vi "Main_PIDTune.vi"() -> ()   [LabVIEW 2015]
doc: "View output from heater including temperature, heater status, temp set point, heater set, and current PWM output (as controlled by PID)."
uses:
  <vilib>/Instr/_visa.llb/VISA Configure Serial Port (Instr).vi
panel:
  out "concatenated string":string
  in  "PID values Set":dbl[](array[numeric])
  out "PID values":dbl[](array[numeric])
  out "PWM":i32
  out "On/Off Set":bool
  out "Measurement History":waveform(dbl)(graph)
  out "Set Point FB":i32 caption="Temp Set Point (C)"
  out "Heater Status":bool
  out "Temp (C)":dbl
  in  "Set Point (C)":i32 caption="Temp Set Point (C)" min=0 max=40
  in  "Heater":bool
  in  "String":string
  in  "Send":bool
  in  "stop":bool
  out "Time of Read":string
  out "Serial Buffer":string
  in  "VISA resource name":refnum<visa-resource-name>
  # "Fluid Heater Control"
  # "Feedback"
  # "Setpoint"
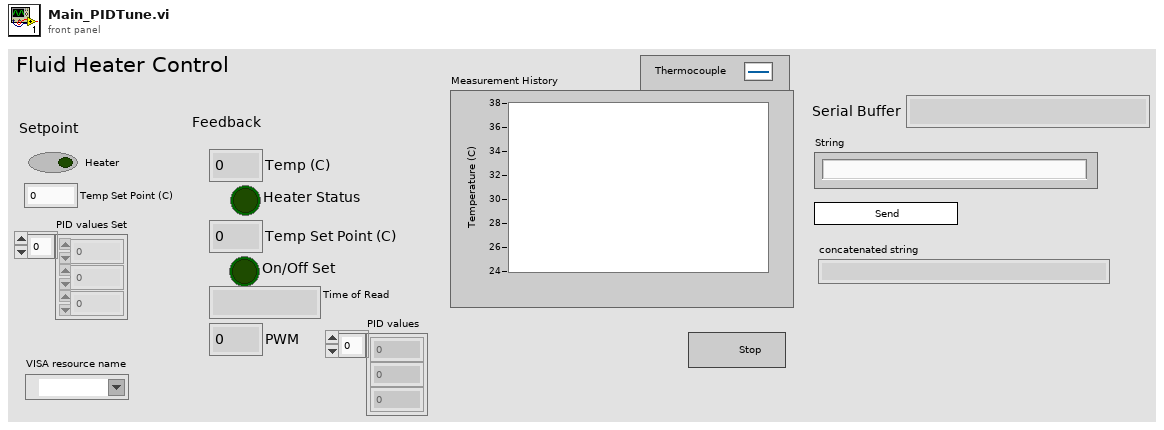
[diagram p1: front panel]
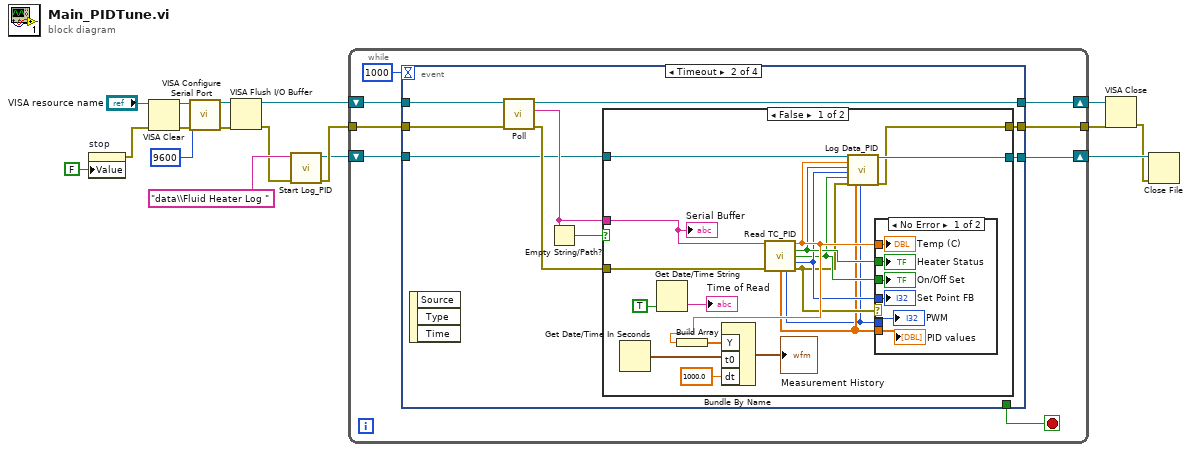
[diagram p0: block diagram]
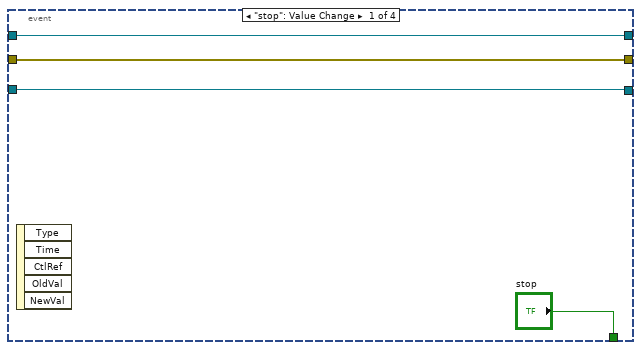
[diagram p2: hidden frame]
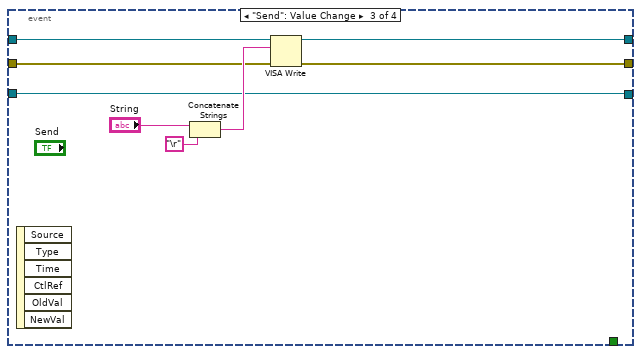
[diagram p5: hidden frame]
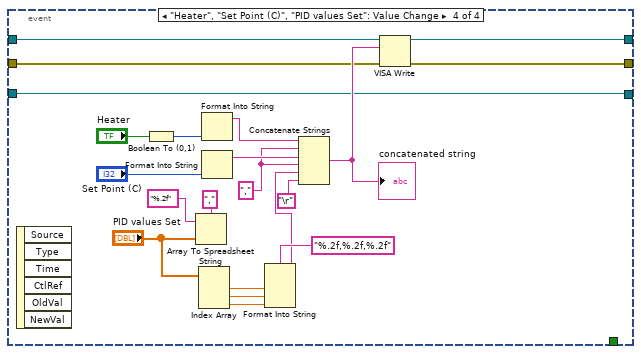
[diagram p6: hidden frame]
diagram:
  n1 = property on="stop" class="Bool (strict)"("Value"=FALSE ("stop")) -> (error out=w8:errorcluster)  [unwired: 2 in, 1 out]
  n2 = VISA Clear(VISA resource name="VISA resource name", error in (no error)=w8) -> (VISA resource name out=w13:refnum<visa-resource-name>, error out=w16:errorcluster)
  n3 = call-poly "VISA Configure Serial Port"("VISA resource name"=w13, "baud rate (9600)"=u32 9600, "error in (no error)"=w16) -> ("VISA resource name out"=w12:refnum<visa-resource-name>, "error out"=w17:errorcluster)  [unwired: 11 in]
  n4 = VISA Flush I/O Buffer(VISA resource name=w12, error in (no error)=w17) -> (VISA resource name out=w11:refnum<visa-resource-name>, error out=w5:errorcluster)  [unwired: 1 in]
  n5 = call "Start Log_PID.vi"("Error In"=w5, "Log Prefix"="data\\Fluid Heater Log ") -> ("Error Out"=w4:errorcluster, "refnum out"=w3:refnum<file>)  [unwired: 8 in]
  n6 = while {
    tunnel: w4 -> [w22]
    shift-right: [w21] -> w10
    shift-left: w11 -> [w23]
    tunnel: [w20] -> w9
    shift-right: [w18] -> w2
    shift-left: w3 -> [w19]
    stop <- w25 stop-if-true
    n7 = event shown="[1] Timeout" {
      selector: _ -> [_ _ _ _]
      dyn-events: _ -> [_ _ _ _]
      timeout: 1000 -> [_ _ _ _]
      tunnel: ["stop" _ _ _] -> w25
      tunnel: w23 -> [w28 w36 w69 w87]
      tunnel: w22 -> [w27 w35 w67 w86]
      tunnel: [w28 w34 w68 w85] -> w21
      tunnel: [w27 w30 w66 w84] -> w20
      tunnel: w19 -> [w26 w32 w65 w83]
      tunnel: [w26 w31 w65 w83] -> w18
      event "stop": Value Change {
        n8 = event-data() -> ()  [unwired: 1 in, 5 out]
      }
      event Timeout {
        n9 = event-data() -> ()  [unwired: 1 in, 3 out]
        n10 = call "Poll.vi"("error in"=w35, "VISA resource name in"=w36) -> ("error out"=w33:errorcluster, "Read"=w38:string, "VISA resource name out"=w34:refnum<visa-resource-name>)  [unwired: 7 in]
        n11 = Empty String/Path?(string/path=w38) -> (empty?=w37:bool)
        n12 = case shown="False" w37 {
          tunnel: w38 -> [w54 _]
          tunnel: w33 -> [w53 w63]
          tunnel: w32 -> [w43 w64]
          tunnel: [w42 w64] -> w31
          tunnel: [w41 w63] -> w30
          frame False {
            n13 = Get Date/Time In Seconds() -> (seconds since 1Jan1904=w52:timestamp)
            n14 = Get Date/Time String(want seconds? (F)=TRUE) -> (time string=→"Time of Read":string)  [unwired: 2 in, 1 out]
            n15 = call "Read TC_PID.vi"("read buffer"=w54, "Error In"=w53) -> ("Temp (C)"=w48:dbl, "On/Off Actual"=w47:bool, "On/Off Set"=w45:bool, "Temp Set Point (C)"=w46:i32, "PID values"=w40:dbl[], "PWM"=w39:i32, "Error Out"=w44:errorcluster)  [unwired: 7 in]
            n16 = Build Array(w48) -> (w51:dbl[])
            n17 = Bundle By Name("Y"=w51, "t0"=w52, "dt"=1000.0) -> (→"Measurement History":waveform(dbl))  [unwired: 1 in]
            n18 = call "Log Data_PID.vi"("refnum in"=w43, "Temp (C)"=w48, "Heater Status"=w47, "Set Point FB"=w46, "On/Off Set"=w45, "Error In"=w44, "PID values"=w40, "PWM"=w39) -> ("refnum out"=w42:refnum<file>, "Error Out"=w41:errorcluster)  [unwired: 10 in]
            n19 = case shown="No Error" w44 {
              tunnel: w48 -> [w62 _]
              tunnel: w47 -> [w61 _]
              tunnel: w46 -> [w60 _]
              tunnel: w45 -> [w59 _]
              tunnel: [w58 _] -> _
              tunnel: w39 -> [w58 _]
              tunnel: w40 -> [w57 _]
              frame No Error {
                "Temp (C)" <- w62
                "Heater Status" <- w61
                "Set Point FB" <- w60
                "On/Off Set" <- w59
                "PWM" <- w58
                "PID values" <- w57
              }
              frame Error {
              }
            }
            "Serial Buffer" <- w54
          }
          frame True {
          }
        }
      }
      event "Send": Value Change {
        n20 = event-data() -> ()  [unwired: 1 in, 6 out]
        n21 = Concatenate Strings("String", "\r") -> (w70:string)
        n22 = VISA Write(VISA resource name=w69, write buffer=w70, error in (no error)=w67) -> (VISA resource name out=w68:refnum<visa-resource-name>, error out=w66:errorcluster)  [unwired: 1 out]
      }
      event "Heater", "Set Point (C)", "PID values Set": Value Change {
        w80 = ","
        n23 = event-data() -> ()  [unwired: 1 in, 6 out]
        n24 = Boolean To (0,1)(Boolean="Heater") -> (0, 1=w90:i16)
        n25 = Array To Spreadsheet String(delimiter (Tab)=",", array="PID values Set", 3:"%.2f" ("format string")) -> ()  [unwired: 1 out]
        n26 = Index Array(array="PID values Set") -> (element #1=w77:dbl, element #2=w76:dbl, element #3=w75:dbl)  [unwired: 3 in]
        n27 = Format Into String(w90) -> (resulting string=w88:string)  [unwired: 3 in, 1 out]
        n28 = Format Into String("Set Point (C)") -> (resulting string=w89:string)  [unwired: 3 in, 1 out]
        n29 = Format Into String(format string="%.2f,%.2f,%.2f", w77, w76, w75) -> (resulting string=w73:string)  [unwired: 2 in, 1 out]
        n30 = Concatenate Strings(w88, w80, w89, w80, w73, "\r") -> (w93:string)
        "concatenated string" <- w93
        n31 = VISA Write(VISA resource name=w87, write buffer=w93, error in (no error)=w86) -> (VISA resource name out=w85:refnum<visa-resource-name>, error out=w84:errorcluster)  [unwired: 1 out]
      }
    }
  }
  n32 = VISA Close(VISA resource name=w10, error in (no error)=w9) -> (error out=w1:errorcluster)
  n33 = Close File(refnum=w2, error in=w1) -> ()  [unwired: 2 out]
